vi "Dialog Get Team Number.vi"() -> (1 "Team Number":string caption="Password")   [LabVIEW 2023]
doc: "Displays a standard dialog box that prompts users to enter information, such as a user name and password.\n--------------------\n\nThis Express VI is configured as follows:\n\nMessage to Display to the User:Please enter the password\nThe inputs are: \nText Entry Box: Password"
uses:
  <vilib>/event_ctls.llb/eventvkey.ctl
panel:
  in  "Tab Control":enum32{"Page 1", "Page 2"}(tab)
  in  "Enter":bool
  in  "Team Number":string caption="Password"
  in  "Server IP Address":string="roboRIO-141-FRC.local"
  # "Enter Team Number"
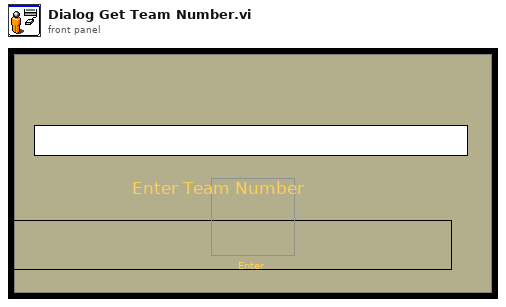
[diagram p1: front panel]
types:
  T1 = typedef "eventvkey.ctl" = enum16{"ASCII", "Enter", "Return", "Shift", "Ctrl", "Alt", "Cmd", "Opt", "Caps", "NumLock", "Clear", "Break", "Up", "Down", "Left", "Right", "Insert", "Delete", "Home", "End", "PageUp", "PageDown", "Escape", "Help", "Pause", "ScrollLock", "F1", "F2", "F3", "F4", "F5", "F6", "F7", "F8", "F9", "F10", "F11", "F12", "F13", "F14", "F15", "F16", "F17", "F18", "F19", "F20", "F21", "F22", "F23", "F24", "Play", "VolumeUp", "VolumeDown", "Mute", "Two Byte Char"}
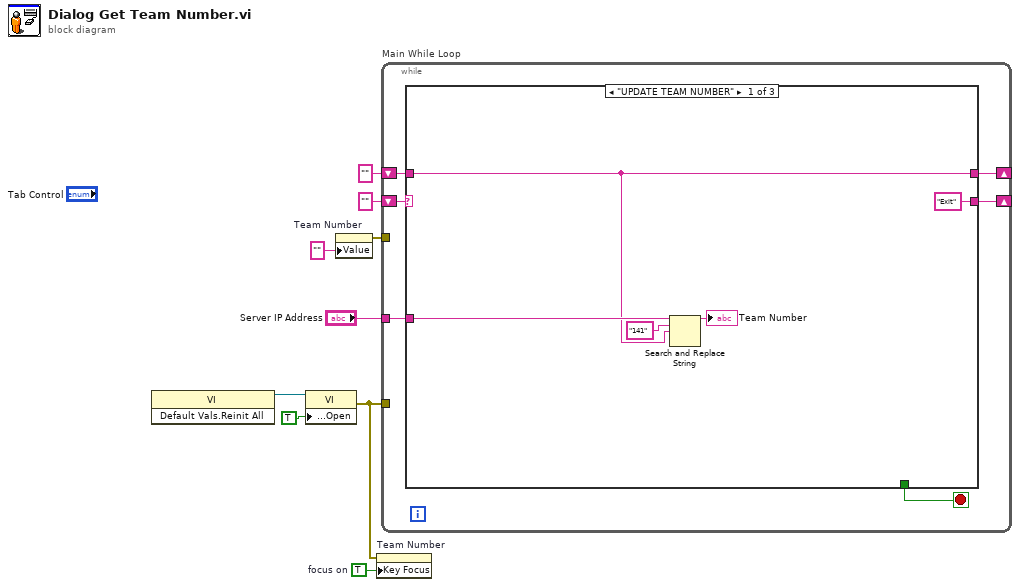
[diagram p0: block diagram]
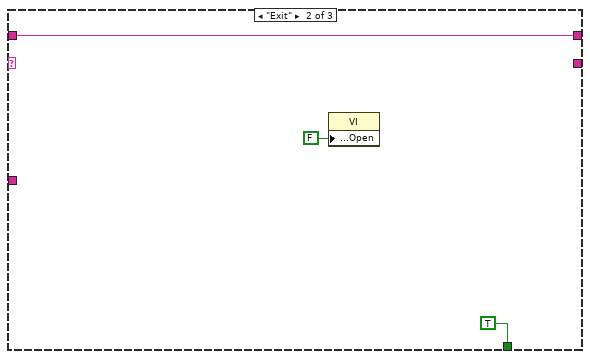
[diagram p2: hidden frame]
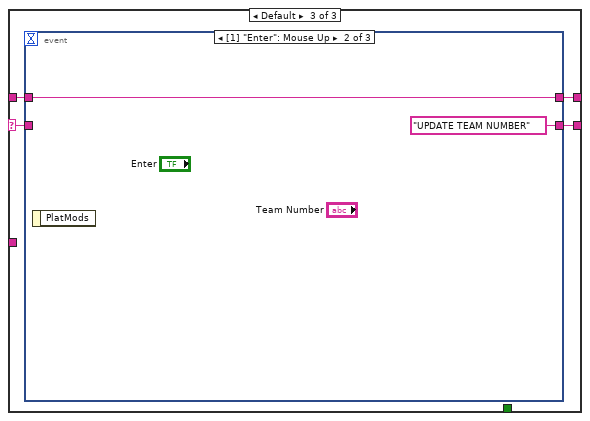
[diagram p3: hidden frame]
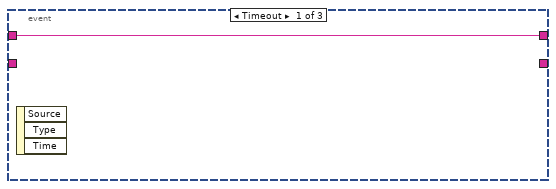
[diagram p4: hidden frame]
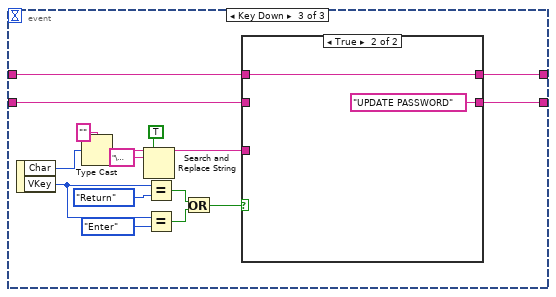
[diagram p5: hidden frame]
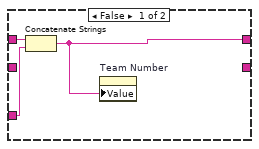
[diagram p6: hidden frame]
diagram:
  w7 = TRUE  # focus on
  n1 = invoke class="VI" method="Default Vals.Reinit All"() -> (reference out=w8:refnum<vi>)  [unwired: 3 in, 2 out]
  n2 = property class="VI"(reference=w8, "Front Panel Window:Open"=TRUE) -> (error out=w6:errorcluster)  [unwired: 1 in, 1 out]
  n3 = property on="Team Number" class="Str"("Value"="" ("Password in")) -> (error out=w2:errorcluster)  [unwired: 2 in, 1 out]
  n4 = property on="Team Number" class="Str"(error in=w6, "Key Focus"=w7) -> ()  [unwired: 1 in, 2 out]
  n5 = while "Main While Loop" {
    tunnel: w6 -> [_]
    shift-right: [w13] -> _
    shift-left: "" -> [w14]
    shift-right: [w11] -> _
    shift-left: "" -> [w12]
    tunnel: w2 -> [_]
    tunnel: "Server IP Address" -> [w10]
    stop <- w15 stop-if-true
    n6 = case shown="\"UPDATE TEAM NUMBER\"" w14 {
      selector: w14 -> [_ _ w27]
      tunnel: [_ TRUE _] -> w15
      tunnel: ["Exit" _ w26] -> w13
      tunnel: w12 -> [w16 w22 w25]
      tunnel: [w16 w22 w24] -> w11
      tunnel: w10 -> [w19 _ _]
      frame "UPDATE TEAM NUMBER" {
        n7 = Search and Replace String(input string=w19, search string="141", replace string=w16) -> (result string=→"Team Number":string)  [unwired: 5 in, 3 out]
      }
      frame "Exit" {
        n8 = property class="VI"("Front Panel Window:Open"=FALSE) -> ()  [unwired: 2 in, 2 out]
      }
      frame Default {
        n9 = event shown="[1] \"Enter\": Mouse Up" {
          selector: _ -> [_ _ _]
          dyn-events: _ -> [_ _ _]
          timeout: _ -> [_ _ _]
          tunnel: w27 -> [_ _ w40]
          tunnel: [_ "UPDATE TEAM NUMBER" w39] -> w26
          tunnel: w25 -> [w28 w29 w35]
          tunnel: [w28 w29 w36] -> w24
          event Timeout {
            n10 = event-data() -> ()  [unwired: 1 in, 3 out]
          }
          event "Enter": Mouse Up {
            n11 = event-data() -> ()  [unwired: 1 in, 1 out]
          }
          event Key Down {
            n12 = event-data() -> ("Char"=w38:i16, "VKey"=w44:T1)  [unwired: 1 in]
            n13 = Type Cast(type="", x=w38) -> (*(type *) &x=w34:string)
            n14 = Search and Replace String(replace all?=TRUE ("replace all? (F)"), input string=w34, search string="\u0000") -> (result string=w31:string)  [unwired: 5 in, 3 out]
            n15 = Equal?(x=w44, y=eventvkey."Return") -> (x = y?=w46:bool)
            n16 = Equal?(x=w44, y=eventvkey."Enter") -> (x = y?=w45:bool)
            n17 = Or(x=w46, y=w45) -> (x .or. y?=w41:bool)
            n18 = case shown="True" w41 {
              tunnel: w40 -> [_ _]
              tunnel: [_ "UPDATE PASSWORD"] -> w39
              tunnel: w35 -> [w49 w50]
              tunnel: [w47 w50] -> w36
              tunnel: w31 -> [w48 _]
              frame False {
                n19 = Concatenate Strings(w49, w48) -> (w47:string)
                n20 = property on="Team Number" class="Str"("Value"=w47) -> ()  [unwired: 2 in, 2 out]
              }
              frame True {
              }
            }
          }
        }
      }
    }
  }
